vi "CCI Time to XL.vi"(6 "Time Stamp":timestamp) -> (1 "Zone":string, 2 "XLTime":dbl format="%#.6g")   [LabVIEW 2021]
doc: "<B> VI name</B>\nCCI Time to XL.vi\n\n<B>Function</B>\nThis vi will convert LabVIEW Time Stamp type to a date-time for reporting to a data file in and Excel readable format. The Time Zone information is available as a string e.g. CDT-05:00:00. Additionally, the vi accounts for the Feb 29,1900 Excel bug and synchronizes all LabVIEW dates with Excel dates. It is of Historical note that Microsoft forgot that the year 1900 was not a leap year. While LabVIEW displays a Feb 29 1900 date it CANNOT be selected.\n\n<B>Inputs</B>\nTime Stamp\n\n<B>Outputs</B>\nXL Time\nZone\n\n<B>Author</B>\nCCI\nJ. Bohrer\n13 Apr 2009\n\n<B>Rev</B>\n16 Jan 2009\nJJB\nUprev to 2009f3\nAdded section to code around the Excel 29 Feb 1900 bug"
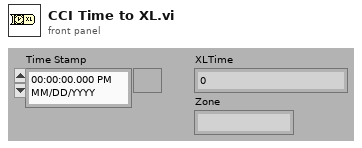
[diagram p1: front panel]
types:
  T1 = typedef "LVDateTimeRec.ctl" = cluster{"fractional second":dbl, "second":i32, "minute":i32, "hour":i32, "day of month":i32, "month":i32, "year":i32, "day of week":i32, "day of year":i32, "DST":i32}
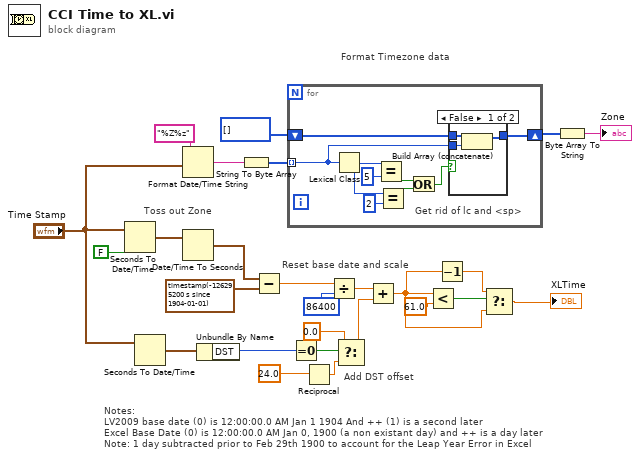
[diagram p0: block diagram]
diagram:
  # "Notes:\nLV2009 base date (0) is 12:00:00.0 AM Jan 1 1904 And ++ (1) is a second later\nExcel Base Date (0) is 12:00:00.0 AM Jan 0, 1900 (a non existant day) and ++ is a day later\nNote: 1 day subtracted prior to Feb 29th 1900 to account for the Leap Year Error in Excel"
  # "Add DST offset"
  # "Reset base date and scale"
  # "Format Timezone data"
  # "Toss out Zone"
  n1 = Seconds To Date/Time(time stamp (now)="Time Stamp", to UTC (F)=FALSE ("is UTC (F)")) -> (date time rec=w16:T1)
  n2 = Seconds To Date/Time(time stamp (now)="Time Stamp") -> (date time rec=w14:T1)  [unwired: 1 out]
  n3 = Format Date/Time String(time format string (%c)="%Z%z", seconds (now)="Time Stamp") -> (date/time string=w24:string)  [unwired: 1 out]
  n4 = Date/Time To Seconds(2:w16) -> (0:w19:timestamp)  [unwired: 1 out]
  n5 = Unbundle By Name(w14) -> ("DST"=w13:i32)
  n6 = String To Byte Array(string=w24) -> (unsigned byte array=w23:u8[])
  n7 = Subtract(x=w19, y=timestamp(-126295200 s since 1904-01-01) ("time stamp 2")) -> (x-y=w18:dbl)
  n8 = for {
    tunnel: w23 -> [w32] mode=indexing
    shift-right: [w34] -> w21
    shift-left: u8[] [] -> [w33]
    # "Get rid of lc and <sp>"
    n9 = Lexical Class(1:w32) -> (0:w27:i16)
    n10 = Equal?(x=w27, y=i16 5) -> (x = y?=w29:bool)
    n11 = Equal?(x=w27, y=i16 2) -> (x = y?=w28:bool)
    n12 = Or(x=w29, y=w28) -> (x .or. y?=w30:bool)
    n13 = case shown="False" w30 {
      tunnel: [w38 w39] -> w34
      tunnel: w33 -> [w37 w39]
      tunnel: w32 -> [w36 _]
      frame False {
        n14 = Build Array (concatenate)(w37, w36) -> (w38:u8[])
      }
      frame True {
      }
    }
  }
  n15 = Equal To 0?(x=w13) -> (x = 0?=w12:bool)
  n16 = Reciprocal(x=24.0 ("f")) -> (1/x=w9:dbl)
  n17 = Divide(x=w18, y=86400) -> (x/y=w7:dbl)
  n18 = Select(t=0.0, s=w12, f=w9) -> (s? t:f=w6:dbl)
  n19 = Add(x=w7, y=w6) -> (x+y=w2:dbl)
  n20 = Less?(x=w2, y=61.0) -> (x < y?=w4:bool)
  n21 = Decrement(x=w2) -> (x-1=w1:dbl)
  n22 = Select(t=w1, s=w4, f=w2) -> (s? t:f=→"XLTime":dbl)
  n23 = Byte Array To String(unsigned byte array=w21) -> (string=→"Zone":string)
